vi "Get Copilot Notifcations.vi"(8 "Error In":errorcluster) -> (0 "error out":errorcluster, 2 "timed out?":bool, 3 "Notification":string)   [LabVIEW 2014]
doc: "Dequeues errors for processing\n\nThis VI will block untill an error appears in the Copilot queue."
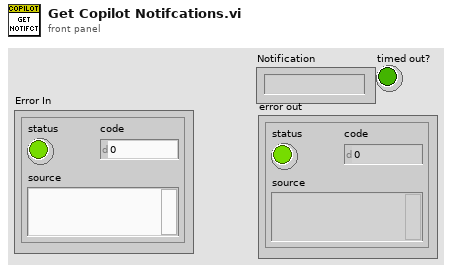
[diagram p1: front panel]
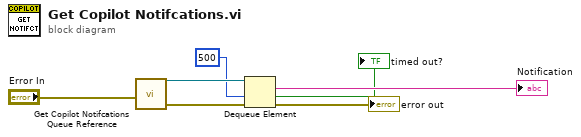
[diagram p0: block diagram]
diagram:
  n1 = call "Get Copilot Notifcations Queue Reference.vi"("Error In"="Error In") -> ("Error Out"=w5:errorcluster, "Co Pilot Notifications Queue Out"=w6:refnum<queue>)  [unwired: 9 in]
  n2 = Dequeue Element(queue=w6, timeout in ms (-1)=500, error in (no error)=w5) -> (element=→"Notification":string, timed out?=→"timed out?":bool, error out=→"error out":errorcluster)  [unwired: 1 out]
